vi "EMS.vi"() -> ()   [LabVIEW 2015, in "Test EMS.lvlib"]
uses:
  Test EMS.lvlib
  EMS state.ctl
  Utilities/Message Strings.llb/Message String Utilities.lvlib
panel:
  out "Status":string
  out "final state":T1
  out "error out":errorcluster
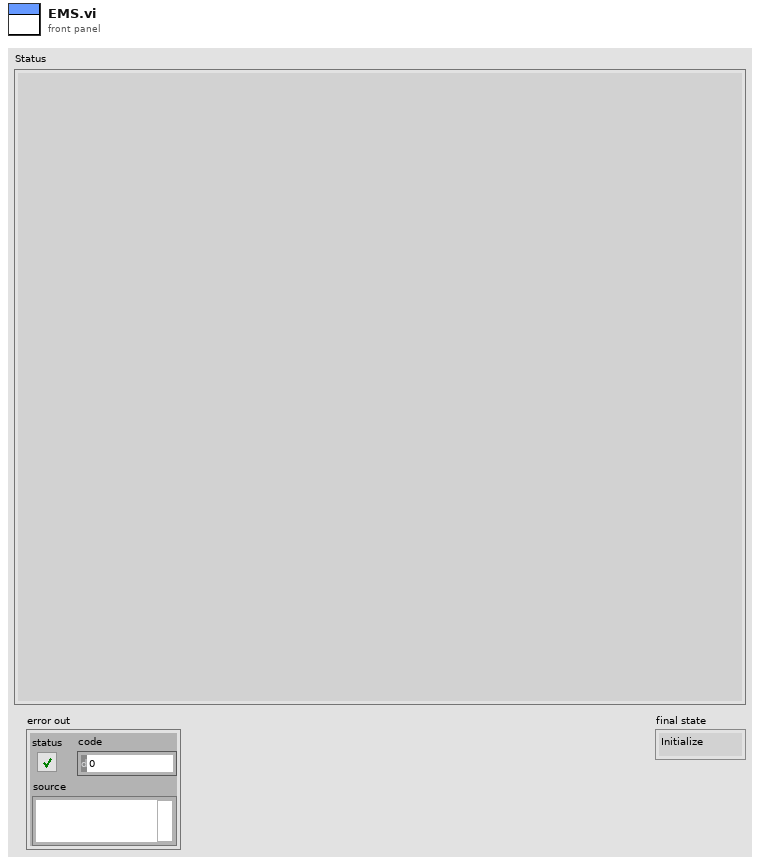
[diagram p1: front panel]
types:
  T1 = typedef "Test EMS.lvlib/EMS state.ctl" = enum16{"Initialize", "Send Files", "Load IEDs", "Set Island Control", "Set PCC", "Activate", "Take Measurements", "Set Setpoints", "Shutdown"}
  T2 = enum16{"big-endian, network order", "native, host order", "little-endian"}
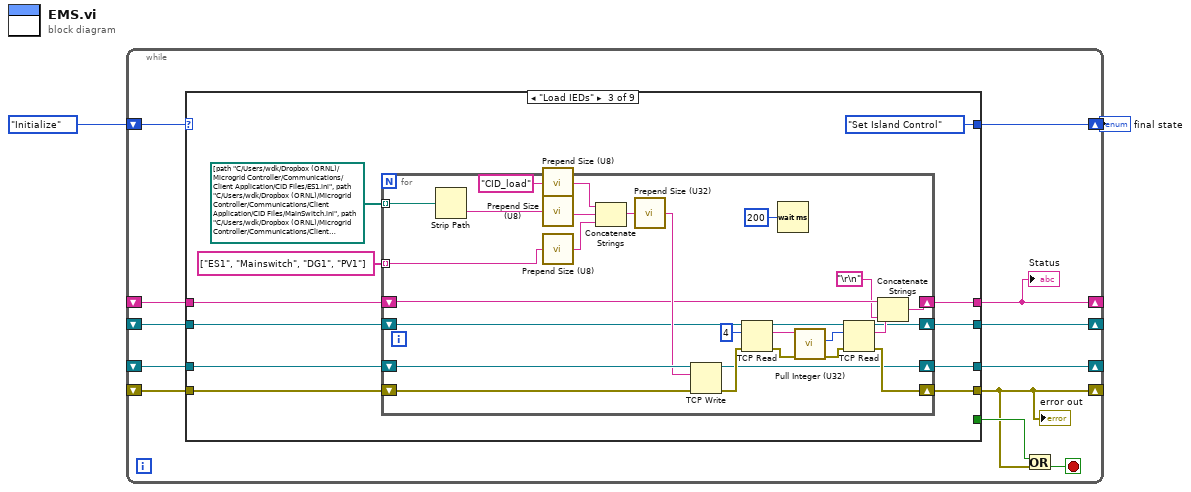
[diagram p0: block diagram]
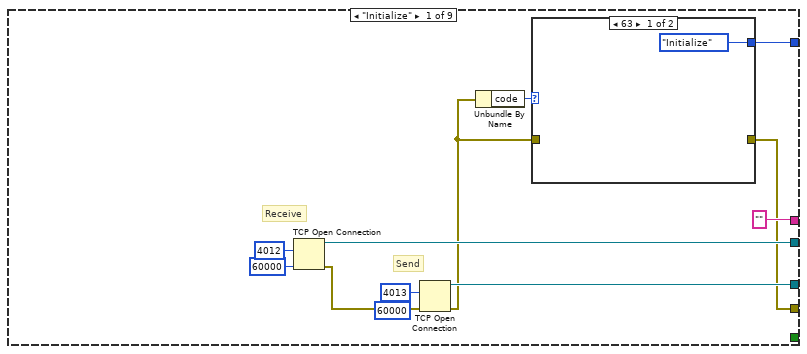
[diagram p2: hidden frame]
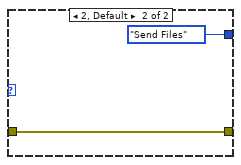
[diagram p3: hidden frame]
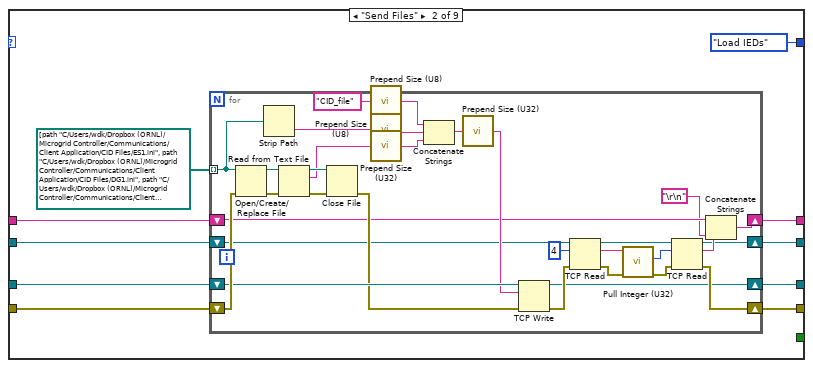
[diagram p4: hidden frame]
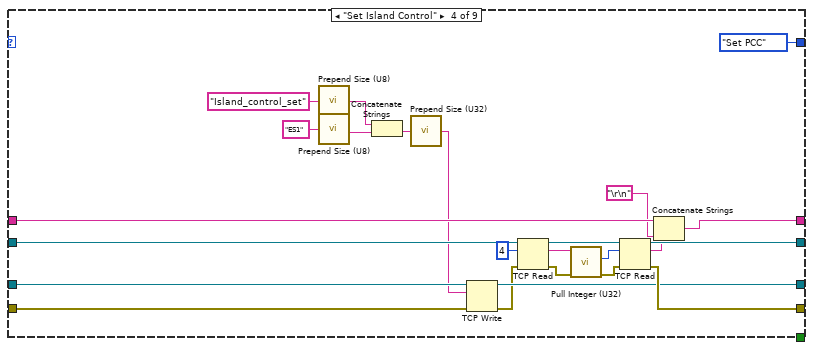
[diagram p5: hidden frame]
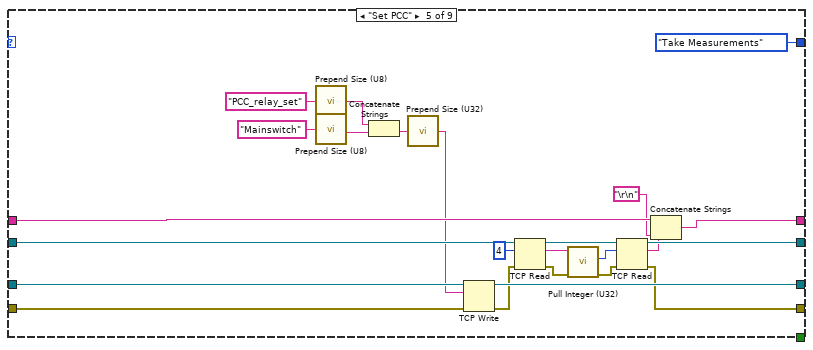
[diagram p6: hidden frame]
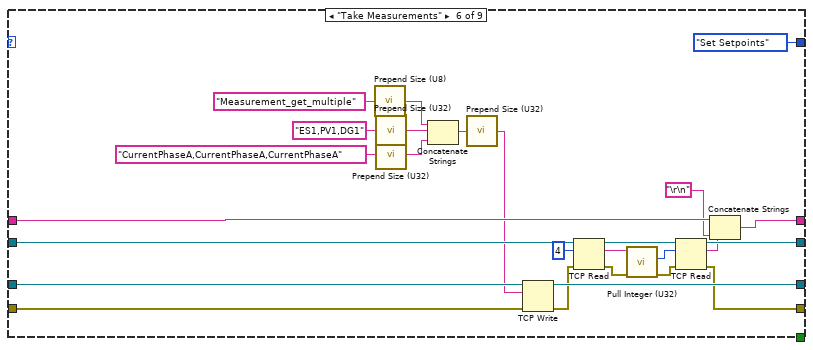
[diagram p7: hidden frame]
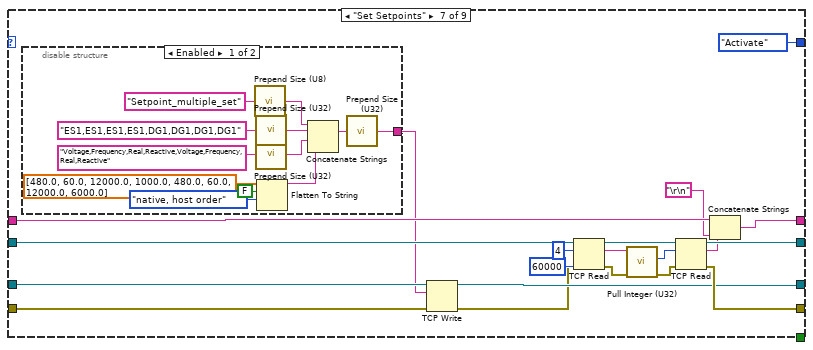
[diagram p8: hidden frame]
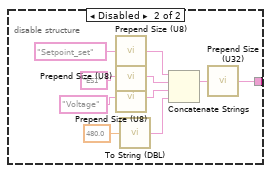
[diagram p9: hidden frame]
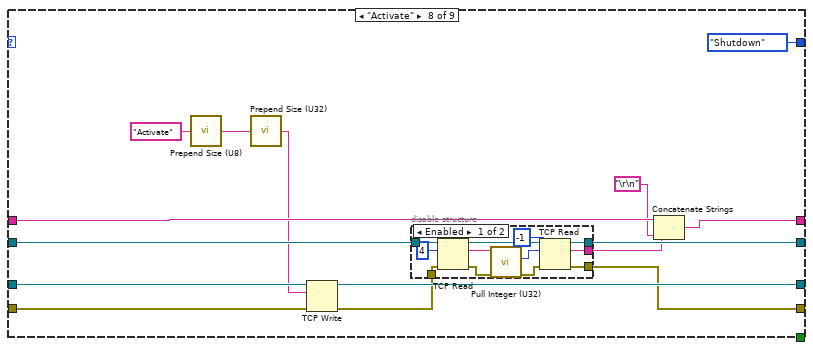
[diagram p10: hidden frame]
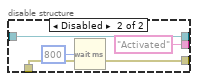
[diagram p11: hidden frame]
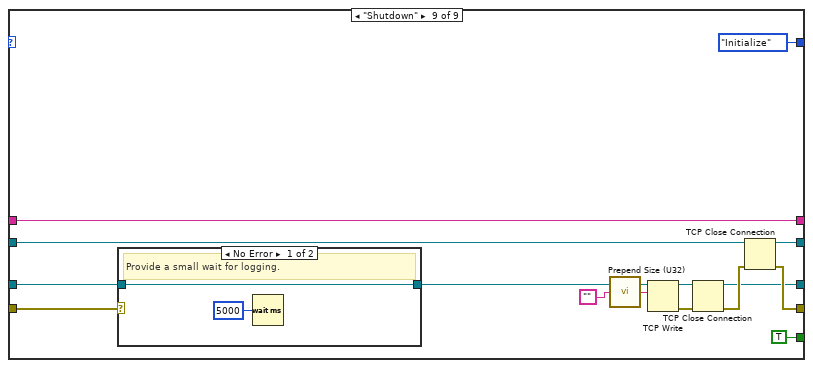
[diagram p12: hidden frame]
diagram:
  n1 = while {
    shift-right: [w9] -> w1
    shift-left: EMS_state."Initialize" -> [w14]
    shift-right: [w13] -> _
    shift-left: _ -> [w10]
    shift-right: [w12] -> _
    shift-left: _ -> [w11]
    shift-right: [w3] -> _
    shift-left: _ -> [w8]
    shift-right: [w6] -> _
    shift-left: _ -> [w7]
    stop <- w5 stop-if-true
    n2 = case shown="\"Load IEDs\"" w14 {
      tunnel: [w23 w33 w74 w126 w149 w175 w184 w232 w264] -> w13
      tunnel: [w22 w32 w75 w125 w150 w176 w196 w233 w263] -> w12
      tunnel: [w15 w31 w73 w127 w148 w174 w195 w231 w265] -> w3
      tunnel: w11 -> [_ w36 w79 w130 w154 w180 w200 w237 w267]
      tunnel: w10 -> [_ w37 w78 w129 w153 w179 w199 w236 w258]
      tunnel: [w21 EMS_state."Load IEDs" EMS_state."Set Island Control" EMS_state."Set PCC" EMS_state."Take Measurements" EMS_state."Set Setpoints" EMS_state."Activate" EMS_state."Shutdown" EMS_state."Initialize"] -> w9
      tunnel: w8 -> [_ w38 w77 w128 w152 w178 w198 w235 w259]
      tunnel: w7 -> [_ w35 w80 w131 w155 w181 w201 w238 w262]
      tunnel: ["" ("Status") w34 w76 w124 w151 w177 w197 w234 w262] -> w6
      tunnel: [_ _ _ _ _ _ _ _ TRUE] -> w4
      frame "Initialize" {
        # "Receive"
        # "Send"
        n3 = TCP Open Connection(remote port or service name=u16 4012, timeout ms (60000)=60000) -> (connection ID=w22:refnum<k5>, error out=w24:errorcluster)  [unwired: 3 in]
        n4 = TCP Open Connection(remote port or service name=u16 4013, timeout ms (60000)=60000, error in (no error)=w24) -> (connection ID=w23:refnum<k5>, error out=w16:errorcluster)  [unwired: 2 in]
        n5 = Unbundle By Name(w16) -> ("code"=w17:i32)
        n6 = case shown="63" w17 {
          tunnel: [EMS_state."Initialize" EMS_state."Send Files"] -> w21
          tunnel: w16 -> [_ w28]
          tunnel: [_ w28] -> w15
          frame 63 {
          }
          frame 2, Default {
          }
        }
      }
      frame "Send Files" {
        n7 = for {
          shift-right: [w48] -> w31
          shift-left: w38 -> [w66]
          tunnel: path[] [path "C:/Users/wdk/Dropbox (ORNL)/Microgrid Controller/Communications/Client Application/CID Files/ES1.ini", path "C:/Users/wdk/Dropbox (ORNL)/Microgrid Controller/Communications/Client Application/CID Files/DG1.ini", path "C:/Users/wdk/Dropbox (ORNL)/Microgrid Controller/Communications/Client Application/CID Files/MainSwitch.ini", path "C:/Users/wdk/Dropbox (ORNL)/Microgrid Controller/Communications/Client Application/CID Files/PV1.ini"] -> [w42] mode=indexing
          shift-right: [w47] -> w34
          shift-left: w35 -> [w46]
          shift-right: [w43] -> w32
          shift-left: w36 -> [w50]
          shift-right: [w44] -> w33
          shift-left: w37 -> [w59]
          n8 = Open/Create/Replace File(file path (use dialog)=w42, error in=w66) -> (refnum out=w70:refnum<file>, error out=w69:errorcluster)  [unwired: 4 in, 1 out]
          n9 = Strip Path(path=w42) -> (name=w41:string)  [unwired: 1 out]
          n10 = Read from Text File(file (use dialog)=w70, error in=w69) -> (refnum out=w68:refnum<file>, text=w65:string, error out=w67:errorcluster)  [unwired: 2 in, 1 out]
          n11 = Close File(refnum=w68, error in=w67) -> (error out=w58:errorcluster)  [unwired: 1 out]
          n12 = call "Prepend Size (U8).vi"("String in"="CID_file") -> ("String out"=w61:string)
          n13 = call "Prepend Size (U8).vi"("String in"=w41) -> ("String out"=w64:string)
          n14 = call "Prepend Size (U32).vi"("String in"=w65) -> ("String out"=w63:string)
          n15 = Concatenate Strings(w61, w64, w63) -> (w60:string)
          n16 = call "Prepend Size (U32).vi"("String in"=w60) -> ("String out"=w57:string)
          n17 = TCP Write(connection ID=w59, data in=w57, error in (no error)=w58) -> (connection ID out=w44:refnum<k5>, error out=w49:errorcluster)  [unwired: 1 in, 1 out]
          n18 = TCP Read(connection ID=w50, bytes to read=4, error in (no error)=w49) -> (connection ID out=w54:refnum<k5>, data out=w52:string, error out=w53:errorcluster)  [unwired: 2 in]
          n19 = call "Pull Integer (U32).vi"("error in (no error)"=w53, "String in"=w52) -> ("error out"=w55:errorcluster, "Integer out"=w56:u32)  [unwired: 7 in, 1 out]
          n20 = TCP Read(connection ID=w54, bytes to read=w56, error in (no error)=w55) -> (connection ID out=w43:refnum<k5>, data out=w45:string, error out=w48:errorcluster)  [unwired: 2 in]
          n21 = Concatenate Strings(w46, w45, "\r\n") -> (w47:string)
        }
      }
      frame "Load IEDs" {
        n22 = for {
          shift-right: [w94] -> w73
          shift-left: w77 -> [w86]
          tunnel: path[] [path "C:/Users/wdk/Dropbox (ORNL)/Microgrid Controller/Communications/Client Application/CID Files/ES1.ini", path "C:/Users/wdk/Dropbox (ORNL)/Microgrid Controller/Communications/Client Application/CID Files/MainSwitch.ini", path "C:/Users/wdk/Dropbox (ORNL)/Microgrid Controller/Communications/Client Application/CID Files/DG1.ini", path "C:/Users/wdk/Dropbox (ORNL)/Microgrid Controller/Communications/Client Application/CID Files/PV1.ini"] -> [w88] mode=indexing
          shift-right: [w93] -> w76
          shift-left: w80 -> [w92]
          shift-right: [w89] -> w75
          shift-left: w79 -> [w96]
          shift-right: [w90] -> w74
          shift-left: w78 -> [w104]
          tunnel: string[] ["ES1", "Mainswitch", "DG1", "PV1"] -> [w84] mode=indexing
          n23 = Strip Path(path=w88) -> (name=w87:string)  [unwired: 1 out]
          n24 = call "Prepend Size (U8).vi"("String in"="CID_load") -> ("String out"=w106:string)
          n25 = call "Prepend Size (U8).vi"("String in"=w87) -> ("String out"=w108:string)
          n26 = call "Prepend Size (U8).vi"("String in"=w84) -> ("String out"=w85:string)
          n27 = Concatenate Strings(w106, w108, w85) -> (w105:string)
          n28 = call "Prepend Size (U32).vi"("String in"=w105) -> ("String out"=w103:string)
          n29 = TCP Write(connection ID=w104, data in=w103, error in (no error)=w86) -> (connection ID out=w90:refnum<k5>, error out=w95:errorcluster)  [unwired: 1 in, 1 out]
          n30 = TCP Read(connection ID=w96, bytes to read=4, error in (no error)=w95) -> (connection ID out=w100:refnum<k5>, data out=w98:string, error out=w99:errorcluster)  [unwired: 2 in]
          n31 = Wait (ms)(milliseconds to wait=u32 200) -> ()  [unwired: 1 out]
          n32 = call "Pull Integer (U32).vi"("error in (no error)"=w99, "String in"=w98) -> ("error out"=w101:errorcluster, "Integer out"=w102:u32)  [unwired: 7 in, 1 out]
          n33 = TCP Read(connection ID=w100, bytes to read=w102, error in (no error)=w101) -> (connection ID out=w89:refnum<k5>, data out=w91:string, error out=w94:errorcluster)  [unwired: 2 in]
          n34 = Concatenate Strings(w92, w91, "\r\n") -> (w93:string)
        }
      }
      frame "Set Island Control" {
        n35 = call "Prepend Size (U8).vi"("String in"="Island_control_set") -> ("String out"=w121:string)
        n36 = call "Prepend Size (U8).vi"("String in"="ES1") -> ("String out"=w123:string)
        n37 = Concatenate Strings(w121, w123) -> (w120:string)
        n38 = call "Prepend Size (U32).vi"("String in"=w120) -> ("String out"=w119:string)
        n39 = TCP Write(connection ID=w129, data in=w119, error in (no error)=w128) -> (connection ID out=w126:refnum<k5>, error out=w112:errorcluster)  [unwired: 1 in, 1 out]
        n40 = TCP Read(connection ID=w130, bytes to read=4, error in (no error)=w112) -> (connection ID out=w116:refnum<k5>, data out=w114:string, error out=w115:errorcluster)  [unwired: 2 in]
        n41 = call "Pull Integer (U32).vi"("error in (no error)"=w115, "String in"=w114) -> ("error out"=w117:errorcluster, "Integer out"=w118:u32)  [unwired: 7 in, 1 out]
        n42 = TCP Read(connection ID=w116, bytes to read=w118, error in (no error)=w117) -> (connection ID out=w125:refnum<k5>, data out=w111:string, error out=w127:errorcluster)  [unwired: 2 in]
        n43 = Concatenate Strings(w131, w111, "\r\n") -> (w124:string)
      }
      frame "Set PCC" {
        n44 = call "Prepend Size (U8).vi"("String in"="PCC_relay_set") -> ("String out"=w145:string)
        n45 = call "Prepend Size (U8).vi"("String in"="Mainswitch") -> ("String out"=w147:string)
        n46 = Concatenate Strings(w145, w147) -> (w144:string)
        n47 = call "Prepend Size (U32).vi"("String in"=w144) -> ("String out"=w143:string)
        n48 = TCP Write(connection ID=w153, data in=w143, error in (no error)=w152) -> (connection ID out=w149:refnum<k5>, error out=w136:errorcluster)  [unwired: 1 in, 1 out]
        n49 = TCP Read(connection ID=w154, bytes to read=4, error in (no error)=w136) -> (connection ID out=w140:refnum<k5>, data out=w138:string, error out=w139:errorcluster)  [unwired: 2 in]
        n50 = call "Pull Integer (U32).vi"("error in (no error)"=w139, "String in"=w138) -> ("error out"=w141:errorcluster, "Integer out"=w142:u32)  [unwired: 7 in, 1 out]
        n51 = TCP Read(connection ID=w140, bytes to read=w142, error in (no error)=w141) -> (connection ID out=w150:refnum<k5>, data out=w135:string, error out=w148:errorcluster)  [unwired: 2 in]
        n52 = Concatenate Strings(w155, w135, "\r\n") -> (w151:string)
      }
      frame "Take Measurements" {
        n53 = call "Prepend Size (U8).vi"("String in"="Measurement_get_multiple") -> ("String out"=w172:string)
        n54 = call "Prepend Size (U32).vi"("String in"="ES1,PV1,DG1") -> ("String out"=w159:string)
        n55 = call "Prepend Size (U32).vi"("String in"="CurrentPhaseA,CurrentPhaseA,CurrentPhaseA") -> ("String out"=w158:string)
        n56 = Concatenate Strings(w172, w159, w158) -> (w171:string)
        n57 = call "Prepend Size (U32).vi"("String in"=w171) -> ("String out"=w170:string)
        n58 = TCP Write(connection ID=w179, data in=w170, error in (no error)=w178) -> (connection ID out=w175:refnum<k5>, error out=w163:errorcluster)  [unwired: 1 in, 1 out]
        n59 = TCP Read(connection ID=w180, bytes to read=4, error in (no error)=w163) -> (connection ID out=w167:refnum<k5>, data out=w165:string, error out=w166:errorcluster)  [unwired: 2 in]
        n60 = call "Pull Integer (U32).vi"("error in (no error)"=w166, "String in"=w165) -> ("error out"=w168:errorcluster, "Integer out"=w169:u32)  [unwired: 7 in, 1 out]
        n61 = TCP Read(connection ID=w167, bytes to read=w169, error in (no error)=w168) -> (connection ID out=w176:refnum<k5>, data out=w162:string, error out=w174:errorcluster)  [unwired: 2 in]
        n62 = Concatenate Strings(w181, w162, "\r\n") -> (w177:string)
      }
      frame "Set Setpoints" {
        n63 = disable-structure shown="Enabled" {
          disable-tunnel: [w211 w221] -> w194
          frame Enabled {
            n64 = call "Prepend Size (U8).vi"("String in"="Setpoint_multiple_set") -> ("String out"=w213:string)
            n65 = call "Prepend Size (U32).vi"("String in"="ES1,ES1,ES1,ES1,DG1,DG1,DG1,DG1") -> ("String out"=w208:string)
            n66 = call "Prepend Size (U32).vi"("String in"="Voltage,Frequency,Real,Reactive,Voltage,Frequency,Real,Reactive") -> ("String out"=w207:string)
            n67 = Flatten To String(anything=dbl[] [480.0, 60.0, 12000.0, 1000.0, 480.0, 60.0, 12000.0, 6000.0], prepend array or string size? (T)=FALSE, byte order (0:big-endian, network order)=T2."native, host order") -> (data string=w203:string)  [unwired: 1 in, 2 out]
            n68 = Concatenate Strings(w213, w208, w207, w203) -> (w212:string)
            n69 = call "Prepend Size (U32).vi"("String in"=w212) -> ("String out"=w211:string)
          }
          frame Disabled {
            n70 = call "Prepend Size (U8).vi"("String in"="Setpoint_set") -> ("String out"=w223:string)
            n71 = call "Prepend Size (U8).vi"("String in"="ES1") -> ("String out"=w220:string)
            n72 = call "Prepend Size (U8).vi"("String in"="Voltage") -> ("String out"=w219:string)
            n73 = call "To String (DBL).vi"("Double in"=480.0) -> ("String out"=w215:string)
            n74 = Concatenate Strings(w223, w220, w219, w215) -> (w222:string)
            n75 = call "Prepend Size (U32).vi"("String in"=w222) -> ("String out"=w221:string)
          }
        }
        n76 = TCP Write(connection ID=w199, data in=w194, error in (no error)=w198) -> (connection ID out=w184:refnum<k5>, error out=w183:errorcluster)  [unwired: 1 in, 1 out]
        n77 = TCP Read(connection ID=w200, bytes to read=4, error in (no error)=w183, 9:60000 ("timeout ms (25000)")) -> (connection ID out=w191:refnum<k5>, data out=w189:string, error out=w190:errorcluster)  [unwired: 1 in]
        n78 = call "Pull Integer (U32).vi"("error in (no error)"=w190, "String in"=w189) -> ("error out"=w192:errorcluster, "Integer out"=w193:u32)  [unwired: 7 in, 1 out]
        n79 = TCP Read(connection ID=w191, bytes to read=w193, error in (no error)=w192) -> (connection ID out=w196:refnum<k5>, data out=w187:string, error out=w195:errorcluster)  [unwired: 2 in]
        n80 = Concatenate Strings(w201, w187, "\r\n") -> (w197:string)
      }
      frame "Activate" {
        n81 = call "Prepend Size (U8).vi"("String in"="Activate") -> ("String out"=w226:string)
        n82 = call "Prepend Size (U32).vi"("String in"=w226) -> ("String out"=w229:string)
        n83 = TCP Write(connection ID=w236, data in=w229, error in (no error)=w235) -> (connection ID out=w232:refnum<k5>, error out=w228:errorcluster)  [unwired: 1 in, 1 out]
        n84 = disable-structure shown="Enabled" {
          disable-tunnel: w237 -> [w251 w254]
          disable-tunnel: [w250 w254] -> w233
          disable-tunnel: [w249 w255] -> w231
          disable-tunnel: w228 -> [w242 w255]
          disable-tunnel: [w241 "Activated" ("data out")] -> w227
          frame Enabled {
            n85 = TCP Read(connection ID=w251, bytes to read=4, error in (no error)=w242) -> (connection ID out=w246:refnum<k5>, data out=w244:string, error out=w245:errorcluster)  [unwired: 2 in]
            n86 = call "Pull Integer (U32).vi"("error in (no error)"=w245, "String in"=w244) -> ("error out"=w247:errorcluster, "Integer out"=w248:u32)  [unwired: 7 in, 1 out]
            n87 = TCP Read(connection ID=w246, bytes to read=w248, error in (no error)=w247, 9:-1 ("timeout ms (25000)")) -> (connection ID out=w250:refnum<k5>, data out=w241:string, error out=w249:errorcluster)  [unwired: 1 in]
          }
          frame Disabled {
            n88 = Wait (ms)(milliseconds to wait=u32 800) -> ()  [unwired: 1 out]
          }
        }
        n89 = Concatenate Strings(w238, w227, "\r\n") -> (w234:string)
      }
      frame "Shutdown" {
        n90 = case shown="No Error" w259 {
          tunnel: w258 -> [w272 w273]
          tunnel: [w272 w273] -> w257
          frame No Error {
            # "Provide a small wait for logging."
            n91 = Wait (ms)(milliseconds to wait=u32 5000) -> ()  [unwired: 1 out]
          }
          frame Error {
          }
        }
        n92 = call "Prepend Size (U32).vi"("String in"="") -> ("String out"=w270:string)
        n93 = TCP Write(connection ID=w257, data in=w270) -> (connection ID out=w268:refnum<k5>, error out=w269:errorcluster)  [unwired: 2 in, 1 out]
        n94 = TCP Close Connection(connection ID=w268, error in (no error)=w269) -> (connection ID out=w264:refnum<k5>, error out=w266:errorcluster)  [unwired: 1 in]
        n95 = TCP Close Connection(connection ID=w267, error in (no error)=w266) -> (connection ID out=w263:refnum<k5>, error out=w265:errorcluster)  [unwired: 1 in]
      }
    }
    "Status" <- w6
    "error out" <- w3
    n96 = Or(x=w4, y=w3) -> (x .or. y?=w5:bool)
  }
  "final state" <- w1
